vi "Mian.vi"() -> ()   [LabVIEW 2017]
doc: "本范例演示从计算机内存缓冲区连续重新生成数据的方法。\n\n关于引脚和硬件功能的信息，见设备相关的文档。"
uses:
  <vilib>/DAQmx/write.llb/DAQmx Write (Analog 1D Wfm NChan NSamp).vi
  <vilib>/DAQmx/create/channels.llb/DAQmx Create Channel (AO-Voltage-Basic).vi
  <vilib>/DAQmx/configure/timing.llb/DAQmx Timing (Sample Clock).vi
  <vilib>/DAQmx/miscellaneous.llb/DAQmx Fill In Error Info.vi
  <resource>/objmgr/daqmx.rc
panel:
  out "AO8":waveform(dbl)(graph)
  in  "Electro-optic Modulator Trigger (AO8) Waveform Parameter":T1={"Voltage of Direction1"=0.95, "Voltage of Direction2"=0.62, "Voltage of Direction3"=0.247} {"Voltage of Direction3" format="%0.2p"; "Voltage of Direction2" format="%0.2p"; "Voltage of Direction1" format="%0.2p"}
  out "Real-time Curve":waveform(dbl)[](graph)
  in  "sCMOS Camrea Trigger (AO6) Waveform Parameter":T2={"Type"=2, "Amplitude"=1.65, "Bias"=1.65, "Duty Ratio(%)"=90.0} {"Duty Ratio(%)" format="%0.2p"; "Bias" format="%0.2p"; "Amplitude" format="%0.2p"; "Type" items=["正弦波", "三角波", "方波", "锯齿波"]}
  out "AO6":waveform(dbl)(graph)
  in  "Frequency Coefficient of AO2/AO4":dbl=15.0 format="%#_13g"
  out "AO4":waveform(dbl)(graph)
  out "AO0":waveform(dbl)(graph)
  in  "Piezoelectric translation Stage Trigger (AO4) Waveform Parameter":T3={"Scanning(μm)"=5.0, "Step(μm)"=0.125, "Conversion Ratio(V/μm)"=0.34722, "Waiting Time(ms)"=100.0} {"Waiting Time(ms)" format="%0.2p"; "Conversion Ratio(V/μm)" format="%0.2p"; "Step(μm)" format="%0.2p"; "Scanning(μm)" format="%0.2p"}
  in  "Testing Channel Trigger (AO0) Waveform Parameter":T2={"Type"=2, "Amplitude"=1.5, "Bias"=1.5, "Duty Ratio(%)"=50.0} {"Duty Ratio(%)" format="%0.2p"; "Bias" format="%0.2p"; "Amplitude" format="%0.2p"; "Type" items=["正弦波", "三角波", "方波", "锯齿波"]}
  in  "Digital Micro-mirror Device Trigger (AO2) Waveform Parameter":T4={"Type"=2, "Amplitude"=0.9, "Bias"=0.9, "Duty Ratio(%)"=50.0, "Duty Cycle"=0.03} {"Duty Ratio(%)" format="%0.2p"; "Bias" format="%0.2p"; "Duty Cycle" format="%0.2p"; "Amplitude" format="%0.2p"; "Type" items=["正弦波", "三角波", "方波", "锯齿波"]}
  out "Hits":dbl=5000.0
  out "AO2":waveform(dbl)(graph)
  in  "Sampling Frequency":dbl=10000.0
  in  "Sample Clock source":tag="OnboardClock"
  in  "Maximum Voltage":dbl=10.0
  in  "Minimum Voltage":dbl=-10.0
  in  "Device Channel":tag="Dev3/ao0, Dev3/ao2, Dev3/ao4, Dev3/ao6, Dev3/ao8"
  out "Actucal Sample Frequency":dbl=1000.0 format="%0.2f"
  # "Channel Setting"
  # "Timming and Buffering Setting"
  # "Waveform Setting"
  # "Real-time Output waveform of analog signal"
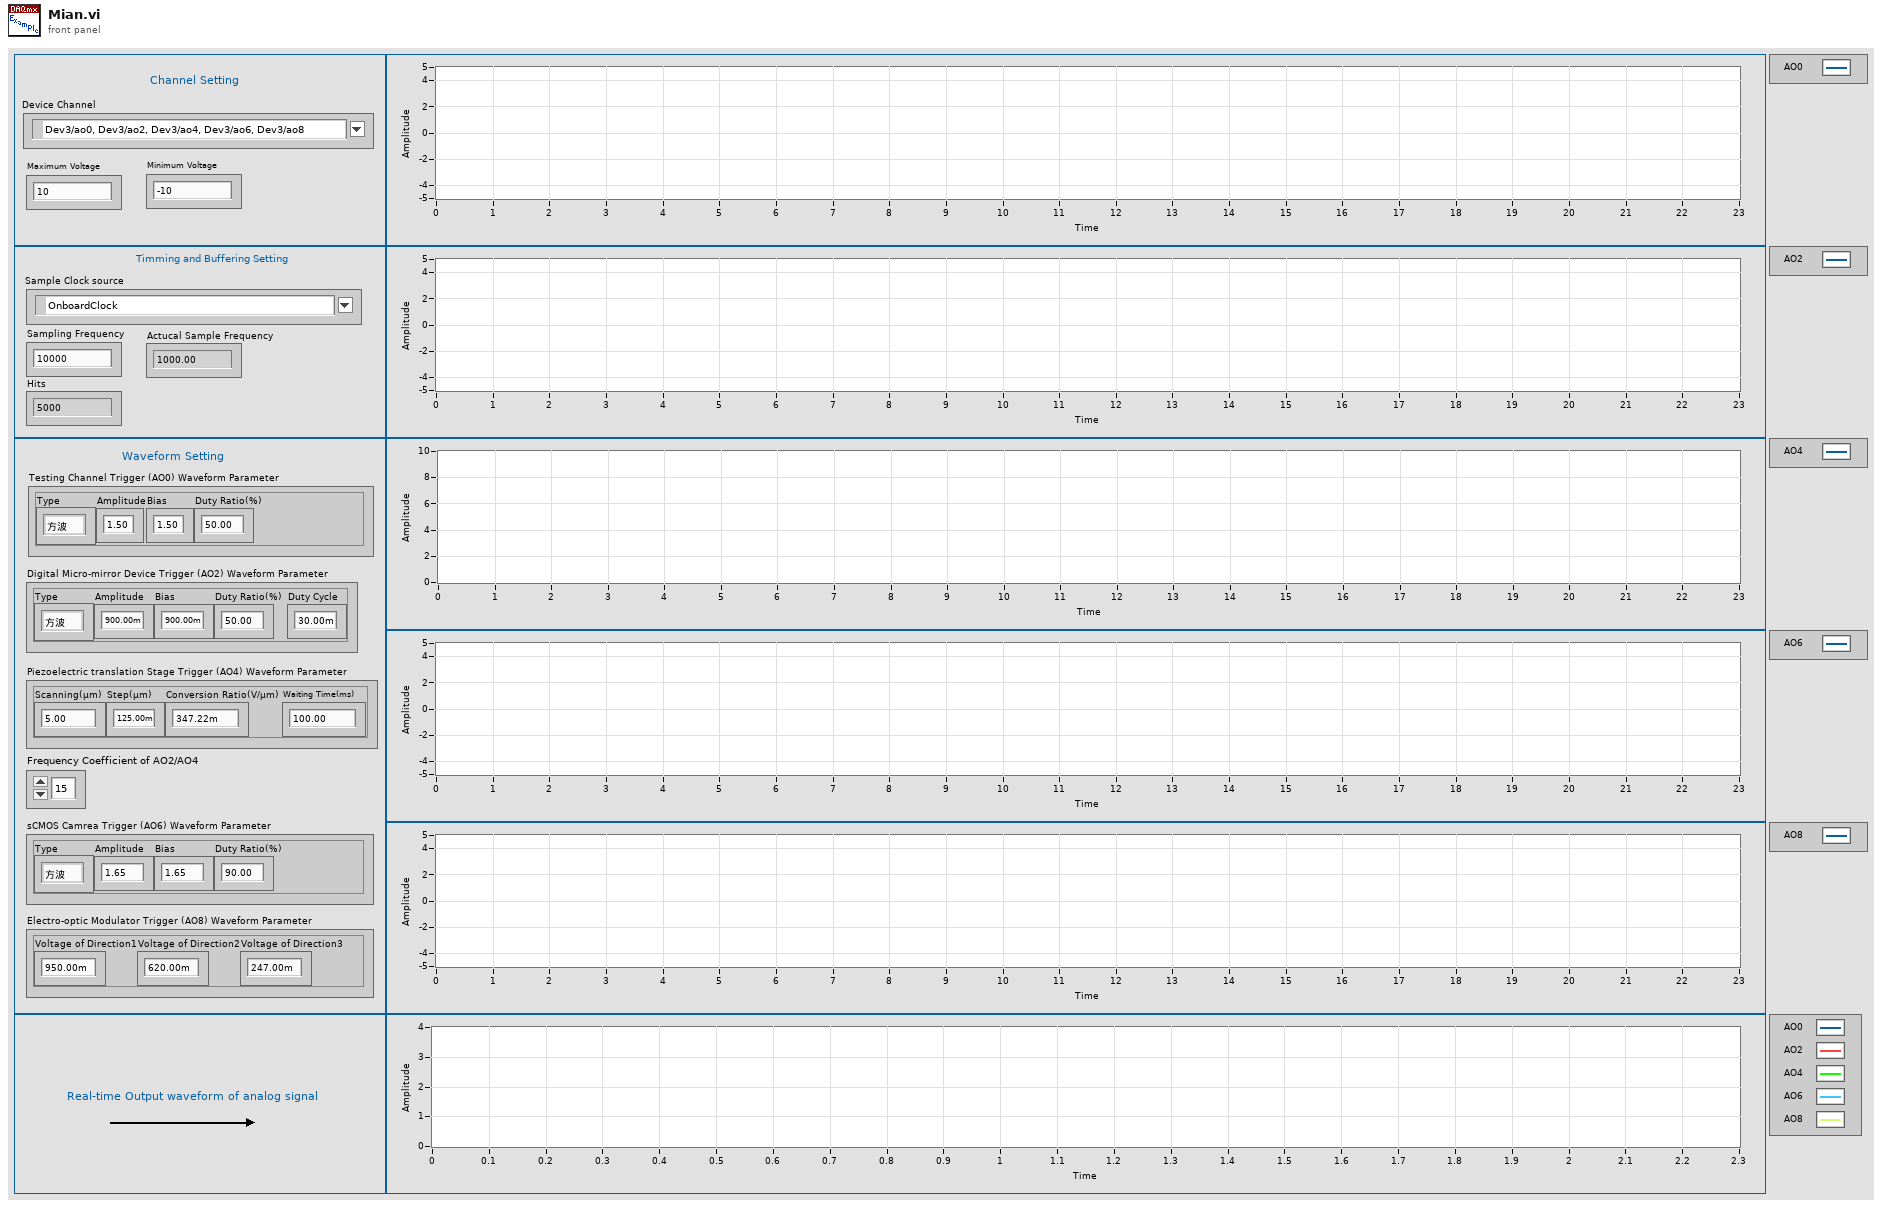
[diagram p1: front panel]
types:
  T1 = cluster{"Voltage of Direction1":dbl, "Voltage of Direction2":dbl, "Voltage of Direction3":dbl}
  T2 = cluster{"Type":u16, "Amplitude":dbl, "Bias":dbl, "Duty Ratio(%)":dbl}
  T3 = cluster{"Scanning(μm)":dbl, "Step(μm)":dbl, "Conversion Ratio(V/μm)":dbl, "Waiting Time(ms)":dbl}
  T4 = cluster{"Type":u16, "Amplitude":dbl, "Bias":dbl, "Duty Ratio(%)":dbl, "Duty Cycle":dbl}
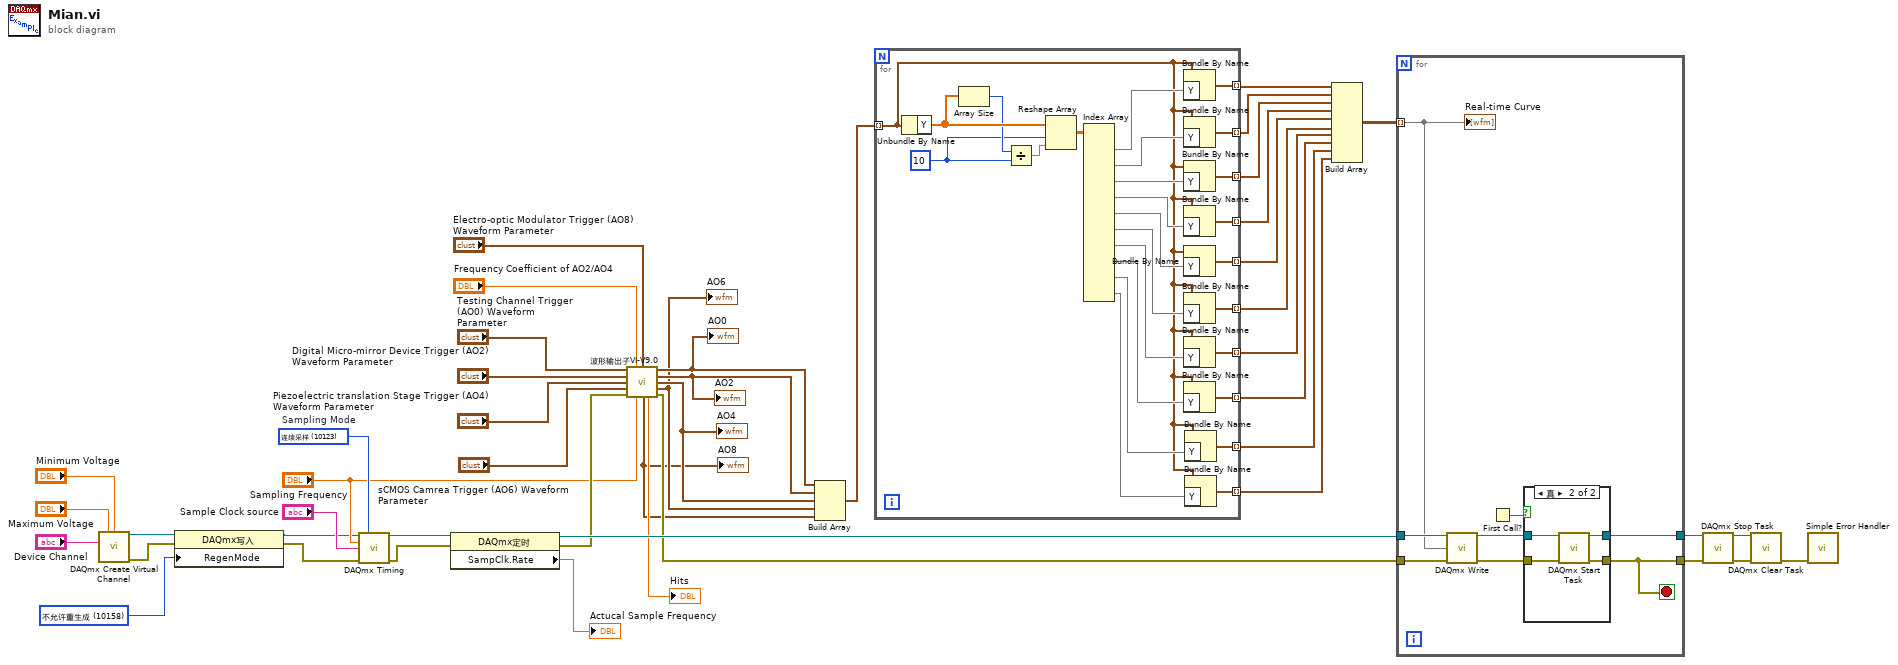
[diagram p0: block diagram]
diagram:
  w16 = 10158 items=["允许重生成"=10097, "不允许重生成"=10158] ("RegenMode")
  w44 = 10123 items=["有限采样"=10178, "连续采样"=10123, "硬件定时单点"=12522]  # Sampling Mode
  n1 = call-poly <vilib>:"DAQmx Create Virtual Channel.vi"("maximum value"="Maximum Voltage", "minimum value"="Minimum Voltage", "physical channels"="Device Channel") -> ("task out"=w20:refnum<k21>, "error out"=w18:errorcluster)  [unwired: 11 in]
  n2 = property class="DAQmx写入"(reference=w20, error in=w18, "RegenMode"=w16) -> (reference out=w19:refnum<k21>, error out=w17:errorcluster)
  n3 = call-poly <vilib>:"DAQmx Timing.vi"("task/channels in"=w19, "sample mode"=w44, "rate"="Sampling Frequency", "source"="Sample Clock source", "error in"=w17) -> ("task out"=w46:refnum<k21>, "error out"=w45:errorcluster)  [unwired: 9 in]
  n4 = property class="DAQmx定时"(reference=w46, error in=w45) -> (reference out=w39:refnum<k21>, error out=w38:errorcluster, "SampClk.Rate"=→"Actucal Sample Frequency":dbl)
  n5 = call "波形输出子VI-V9.0.vi"("AO0波形参数"="Testing Channel Trigger (AO0) Waveform Parameter", "频率比例系数"="Frequency Coefficient of AO2/AO4", "AO8波形参数"="Electro-optic Modulator Trigger (AO8) Waveform Parameter", "AO2波形参数"="Digital Micro-mirror Device Trigger (AO2) Waveform Parameter", "AO4波形参数"="Piezoelectric translation Stage Trigger (AO4) Waveform Parameter", "AO6波形参数"="sCMOS Camrea Trigger (AO6) Waveform Parameter", "Error in"=w38, "采样率"="Sampling Frequency") -> ("AO0"=w28:waveform(dbl), "AO2"=w30:waveform(dbl), "AO4"=w29:waveform(dbl), "AO6"=w26:waveform(dbl), "AO8"=w1:waveform(dbl), "采样数"=→"Hits":dbl, "Error out"=w36:errorcluster)  [unwired: 1 in]
  "AO2" <- w30
  "AO0" <- w28
  "AO4" <- w29
  "AO6" <- w26
  "AO8" <- w1
  n6 = Build Array(w28, w30, w29, w26, w1) -> (w15:waveform(dbl)[])
  n7 = for {
    tunnel: w15 -> [w57] mode=indexing
    tunnel: [w56] -> w13 mode=indexing
    tunnel: [w55] -> w12 mode=indexing
    tunnel: [w54] -> w11 mode=indexing
    tunnel: [w53] -> w10 mode=indexing
    tunnel: [w52] -> w9 mode=indexing
    tunnel: [w51] -> w8 mode=indexing
    tunnel: [w50] -> w7 mode=indexing
    tunnel: [w49] -> w6 mode=indexing
    tunnel: [w48] -> w5 mode=indexing
    tunnel: [w47] -> w4 mode=indexing
    w69 = 10 ("维数大小")
    n8 = Unbundle By Name(w57) -> ("Y"=w72:dbl[])
    n9 = Array Size(array=w72) -> (size(s)=w70:i32)
    n10 = Divide(x=w70, y=w69) -> (x/y=w71:dbl)
    n11 = Reshape Array(w72, w69, w71) -> (w68:dbl[][])
    n12 = Index Array(array=w68) -> (element #1=w67:dbl[], element #2=w66:dbl[], element #3=w65:dbl[], element #4=w64:dbl[], element #5=w63:dbl[], element #6=w62:dbl[], element #7=w61:dbl[], element #8=w60:dbl[], element #9=w59:dbl[], element #10=w58:dbl[])  [unwired: 20 in]
    n13 = Bundle By Name(cluster=w57, "Y"=w67) -> (w56:waveform(dbl))
    n14 = Bundle By Name(cluster=w57, "Y"=w66) -> (w55:waveform(dbl))
    n15 = Bundle By Name(cluster=w57, "Y"=w65) -> (w54:waveform(dbl))
    n16 = Bundle By Name(cluster=w57, "Y"=w64) -> (w53:waveform(dbl))
    n17 = Bundle By Name(cluster=w57, "Y"=w63) -> (w52:waveform(dbl))
    n18 = Bundle By Name(cluster=w57, "Y"=w62) -> (w51:waveform(dbl))
    n19 = Bundle By Name(cluster=w57, "Y"=w61) -> (w50:waveform(dbl))
    n20 = Bundle By Name(cluster=w57, "Y"=w60) -> (w49:waveform(dbl))
    n21 = Bundle By Name(cluster=w57, "Y"=w59) -> (w48:waveform(dbl))
    n22 = Bundle By Name(cluster=w57, "Y"=w58) -> (w47:waveform(dbl))
  }
  n23 = Build Array(w13, w12, w11, w10, w9, w8, w7, w6, w5, w4) -> (w3:waveform(dbl)[][])
  n24 = for {
    tunnel: w3 -> [w74] mode=indexing
    tunnel: w39 -> [w78]
    tunnel: [w76] -> w23
    tunnel: w36 -> [w77]
    tunnel: [w73] -> w22
    stop <- w73 stop-if-true
    n25 = call-poly <vilib>:"DAQmx Write.vi"("task/channels in"=w78, "data"=w74, "error in"=w77) -> ("task out"=w80:refnum<k21>, "error out"=w79:errorcluster)  [unwired: 10 in, 1 out]
    n26 = First Call?() -> (First Call?: T/F=w75:bool)
    n27 = case shown="真" w75 {
      tunnel: w80 -> [w82 w86]
      tunnel: w79 -> [w81 w85]
      tunnel: [w82 w84] -> w76
      tunnel: [w81 w83] -> w73
      frame False {
      }
      frame True {
        n28 = call <vilib>:"DAQmx Start Task.vi"("task/channels in"=w86, "error in"=w85) -> ("task out"=w84:refnum<k21>, "error out"=w83:errorcluster)  [unwired: 12 in]
      }
    }
    "Real-time Curve" <- w74
  }
  n29 = call <vilib>:"DAQmx Stop Task.vi"("task/channels in"=w23, "error in"=w22) -> ("task out"=w25:refnum<k21>, "error out"=w24:errorcluster)  [unwired: 12 in]
  n30 = call <vilib>:"DAQmx Clear Task.vi"("task in"=w25, "error in"=w24) -> ("error out"=w21:errorcluster)  [unwired: 13 in]
  n31 = call <vilib>:"Simple Error Handler.vi"("error in (no error)"=w21) -> ()  [unwired: 4 in, 5 out]
